vi "MapSim.vi"() -> ()   [LabVIEW 2018]
uses:
  <vilib>/imath/engines/lvmath/Plug In/_Char/NIMS_CH_character datatype.ctl
  <vilib>/Analysis/coordinate.llb/2D Cartesian Coordinate Rotation (Scalar).vi
  <vilib>/robotics/Navigation/shared/WorldMap/OccupancyGridWorldMap/NI_Robotics_OccupancyGridWorldMap.lvclass
  C:/Program Files (x86)/National Instruments/LabVIEW 2018/vi.lib/robotics/Navigation/shared/WorldMap/AbstractWorldMap/NI_Robotics_AbstractWorldMap.lvclass
  <vilib>/robotics/Navigation/shared/MapNode/OccupancyGridNode/NI_Robotics_OccupancyGridMapNode.lvclass
  C:/Program Files (x86)/National Instruments/LabVIEW 2018/vi.lib/robotics/Navigation/shared/MapNode/AbstractAstarNode/NI_Robotics_AbstractAstarNode.lvclass
  <vilib>/imath/engines/lvmath2/RunTimeEngine/Managers/WorkSpace/UID Generator.vi
  <vilib>/imath/engines/lvmath/Plug In/_Char/NIMS_CH_String to Character Array.vi
  <vilib>/imath/engines/lvmath2/RunTimeEngine/IndexRead/NIMS V(S).vi
  <instcachedir>/0/NIMS V(S)_0488751826AF41519A22953C041130DC.lvgen/NIMS V(S)_0488751826AF41519A22953C041130DC_003.vi
  <vilib>/imath/engines/lvmath2/RunTimeEngine/RunTimeType/NIMS_RunTimeType_From StrictType (excl LVString).vi
  <instcachedir>/0/NIMS_RunTimeType_From StrictType (excl LVString)_E7E34A65C99947108168652BAD14964D.lvgen/NIMS_RunTimeType_From StrictType (excl LVString)_E7E34A65C99947108168652BAD14964D_000.vi
  <vilib>/imathl/engines/lvmath/Functions/Error Handling/Create Error.vi
  <vilib>/imath/engines/lvmath2/RunTimeEngine/LocalVariableDefStatement/MC_LocalVariableDefStatement_Display.vi
  <vilib>/imath/engines/lvmath2/RunTimeEngine/BuiltInFunctions/acos/NIMS_acos(C).vi
  <instcachedir>/0/NIMS_acos(C)_EB9F8BBCD4F84158BAE4AC9B979C42E8.lvgen/NIMS_acos(C)_EB9F8BBCD4F84158BAE4AC9B979C42E8_001.vi
  <vilib>/imath/engines/lvmath2/RunTimeEngine/Managers/SymbolTable/Clear UID.vi
  <vilib>/imath/engines/lvmath2/RunTimeEngine/NodeEndStatement/NIMS_NodeEndStatement_Output.vi
  <instcachedir>/0/NIMS_NodeEndStatement_Output_53EC0D466D134D7ABD903AC30B43404B.lvgen/NIMS_NodeEndStatement_Output_53EC0D466D134D7ABD903AC30B43404B_001.vi
  <instcachedir>/0/NIMS_NodeEndStatement_Output_53EC0D466D134D7ABD903AC30B43404B.lvgen/NIMS_NodeEndStatement_Output_53EC0D466D134D7ABD903AC30B43404B_011.vi
  <instcachedir>/0/NIMS_NodeEndStatement_Output_53EC0D466D134D7ABD903AC30B43404B.lvgen/NIMS_NodeEndStatement_Output_53EC0D466D134D7ABD903AC30B43404B_009.vi
  <vilib>/imath/engines/lvmath2/RunTimeEngine/ErrorHandling/NIMS_Finalize Error.vi
  <vilib>/imath/engines/lvmath2/RunTimeEngine/BuiltInFunctions/round/NIMS_round(DBL-S).vi
  <vilib>/imath/engines/lvmath2/RunTimeEngine/BuiltInFunctions/char/NIMS_char.vi
  <vilib>/imath/engines/lvmath/Plug In/_Char/NIMS_CH_String CV to Character 2D.vi
  <instcachedir>/0/NIMS_CH_String CV to Character 2D_831D8380D97041D793313BBAC4831DC8.lvgen/NIMS_CH_String CV to Character 2D_831D8380D97041D793313BBAC4831DC8_000.vi
  <instcachedir>/0/NIMS_RunTimeType_From StrictType (excl LVString)_E7E34A65C99947108168652BAD14964D.lvgen/NIMS_RunTimeType_From StrictType (excl LVString)_E7E34A65C99947108168652BAD14964D_001.vi
  <vilib>/imath/engines/lvmath/Plug In/_Char/NIMS_CH_Character 2D to String 1D.vi
  <vilib>/imath/engines/lvmath2/RunTimeSupport/NIMS_Error if Not Equal.vi
  <instcachedir>/0/NIMS_Error if Not Equal_C77461FADD9B4AE6B0EA3ED6E3A6D94D.lvgen/NIMS_Error if Not Equal_C77461FADD9B4AE6B0EA3ED6E3A6D94D_000.vi
  <vilib>/imath/engines/lvmath2/RunTimeEngine/IndexReplace/NIMS M(S,S)=S.vi
  <instcachedir>/0/NIMS M(S,S)=S_5DAF17B45D8A4C8588C7CF468644990A.lvgen/NIMS M(S,S)=S_5DAF17B45D8A4C8588C7CF468644990A_002.vi
  <vilib>/imath/engines/lvmath2/RunTimeEngine/ErrorHandling/NIMS_Create Error From Enums.vi
  <vilib>/imath/engines/lvmath2/RunTimeEngine/RangeToken/NIMS_Range_R2 - Integer.vi
  <instcachedir>/0/NIMS_Range_R2 - Integer_E35B921DECF84AADB7325A02D418BFCC.lvgen/NIMS_Range_R2 - Integer_E35B921DECF84AADB7325A02D418BFCC_000.vi
  <vilib>/imath/engines/lvmath2/RunTimeEngine/CommandStatement/MC_CommandStatement_break.vi
  <vilib>/imath/engines/lvmath2/RunTimeEngine/BuiltInFunctions/min/2 inputs/NIMS_min(RG,RG)-no size check.vi
  <instcachedir>/0/NIMS_min(RG,RG)-no size check_7F67BAB91AFC452D9517D2EA1C8F5F88.lvgen/NIMS_min(RG,RG)-no size check_7F67BAB91AFC452D9517D2EA1C8F5F88_001.vi
  <vilib>/imath/engines/lvmath2/RunTimeEngine/BuiltInFunctions/max/2 inputs/NIMS_max(RG,RG)-no size check.vi
  <instcachedir>/0/NIMS_max(RG,RG)-no size check_F871939977644B7683C1350DCCAD7557.lvgen/NIMS_max(RG,RG)-no size check_F871939977644B7683C1350DCCAD7557_001.vi
  <vilib>/imath/engines/lvmath2/RunTimeEngine/IndexRead/NIMS M(S,S).vi
  <instcachedir>/0/NIMS M(S,S)_AC51E74150A542F7991B9634C66F3096.lvgen/NIMS M(S,S)_AC51E74150A542F7991B9634C66F3096_002.vi
  <instcachedir>/0/NIMS_min(RG,RG)-no size check_7F67BAB91AFC452D9517D2EA1C8F5F88.lvgen/NIMS_min(RG,RG)-no size check_7F67BAB91AFC452D9517D2EA1C8F5F88_002.vi
  <instcachedir>/0/NIMS_min(RG,RG)-no size check_7F67BAB91AFC452D9517D2EA1C8F5F88.lvgen/NIMS_min(RG,RG)-no size check_7F67BAB91AFC452D9517D2EA1C8F5F88_003.vi
  <vilib>/imath/engines/lvmath2/RunTimeEngine/VariableToken/NIMS_VariableToken_CondDefined.vi
  <instcachedir>/0/NIMS_VariableToken_CondDefined_BADDB804EBCA4B86883699DABD34B224.lvgen/NIMS_VariableToken_CondDefined_BADDB804EBCA4B86883699DABD34B224_004.vi
  <vilib>/imath/engines/lvmath/Functions/Error Handling/MergeErrorsWrapper.vi
  <instcachedir>/0/NIMS_NodeEndStatement_Output_53EC0D466D134D7ABD903AC30B43404B.lvgen/NIMS_NodeEndStatement_Output_53EC0D466D134D7ABD903AC30B43404B_012.vi
  <instcachedir>/0/NIMS_NodeEndStatement_Output_53EC0D466D134D7ABD903AC30B43404B.lvgen/NIMS_NodeEndStatement_Output_53EC0D466D134D7ABD903AC30B43404B_013.vi
  <instcachedir>/0/NIMS_NodeEndStatement_Output_53EC0D466D134D7ABD903AC30B43404B.lvgen/NIMS_NodeEndStatement_Output_53EC0D466D134D7ABD903AC30B43404B_016.vi
  <vilib>/imath/engines/lvmath2/RunTimeEngine/Managers/SymbolTable/NIMS_WorkSpace.lvlib
  <vilib>/Analysis/NI_AALPro.lvlib
  <vilib>/robotics/Navigation/NI_Robotics_Navigation .lvlib
panel:
  out "y coordinates":i32[](array[numeric])
  out "x coordinates":i32[](array[numeric])
  out "dy":dbl
  out "dx":dbl
  out "G":i32[][](array[numeric])
  out "dx_char":string[](array[string])
  out "dy_char":string[](array[string])
  in  "QR Data":string
  out "Field":u8[][](array[numeric])
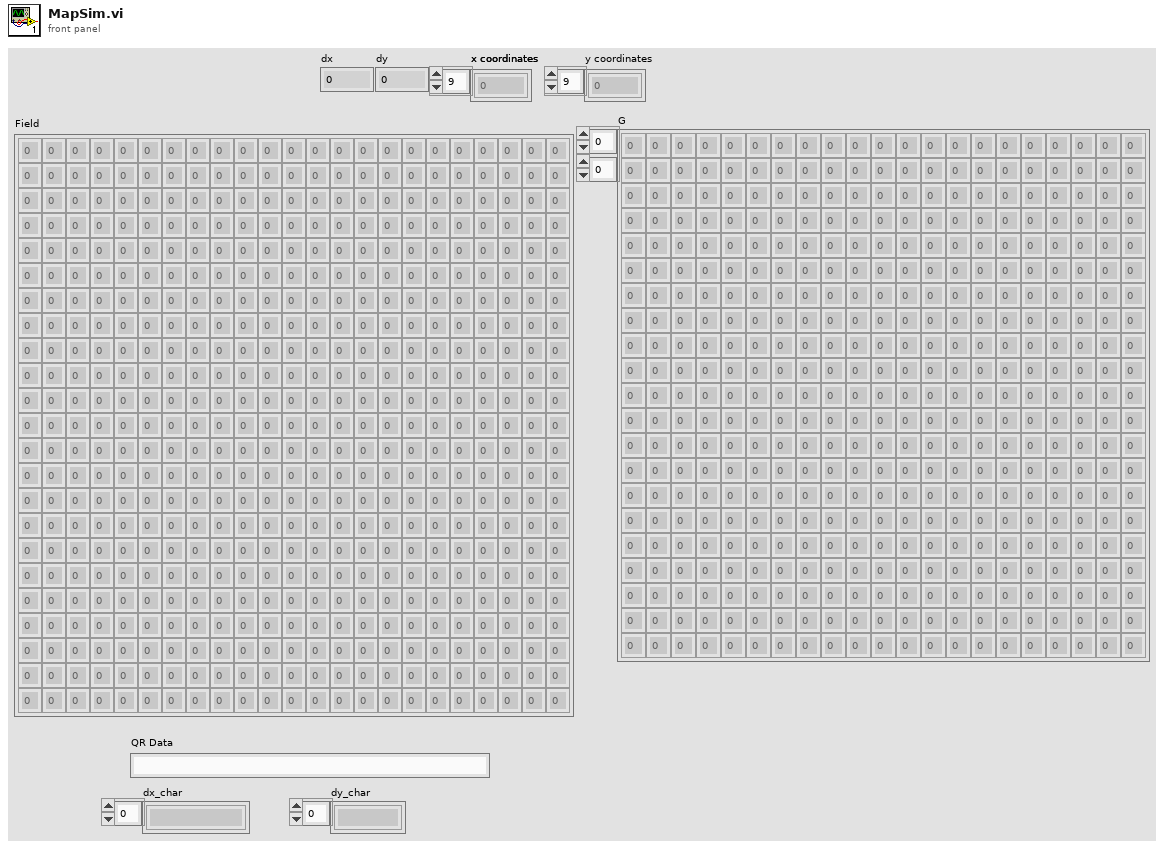
[diagram p1: front panel]
types:
  T1 = typedef "NIMS_CH_character datatype.ctl" = cluster{"Numeric":u8}
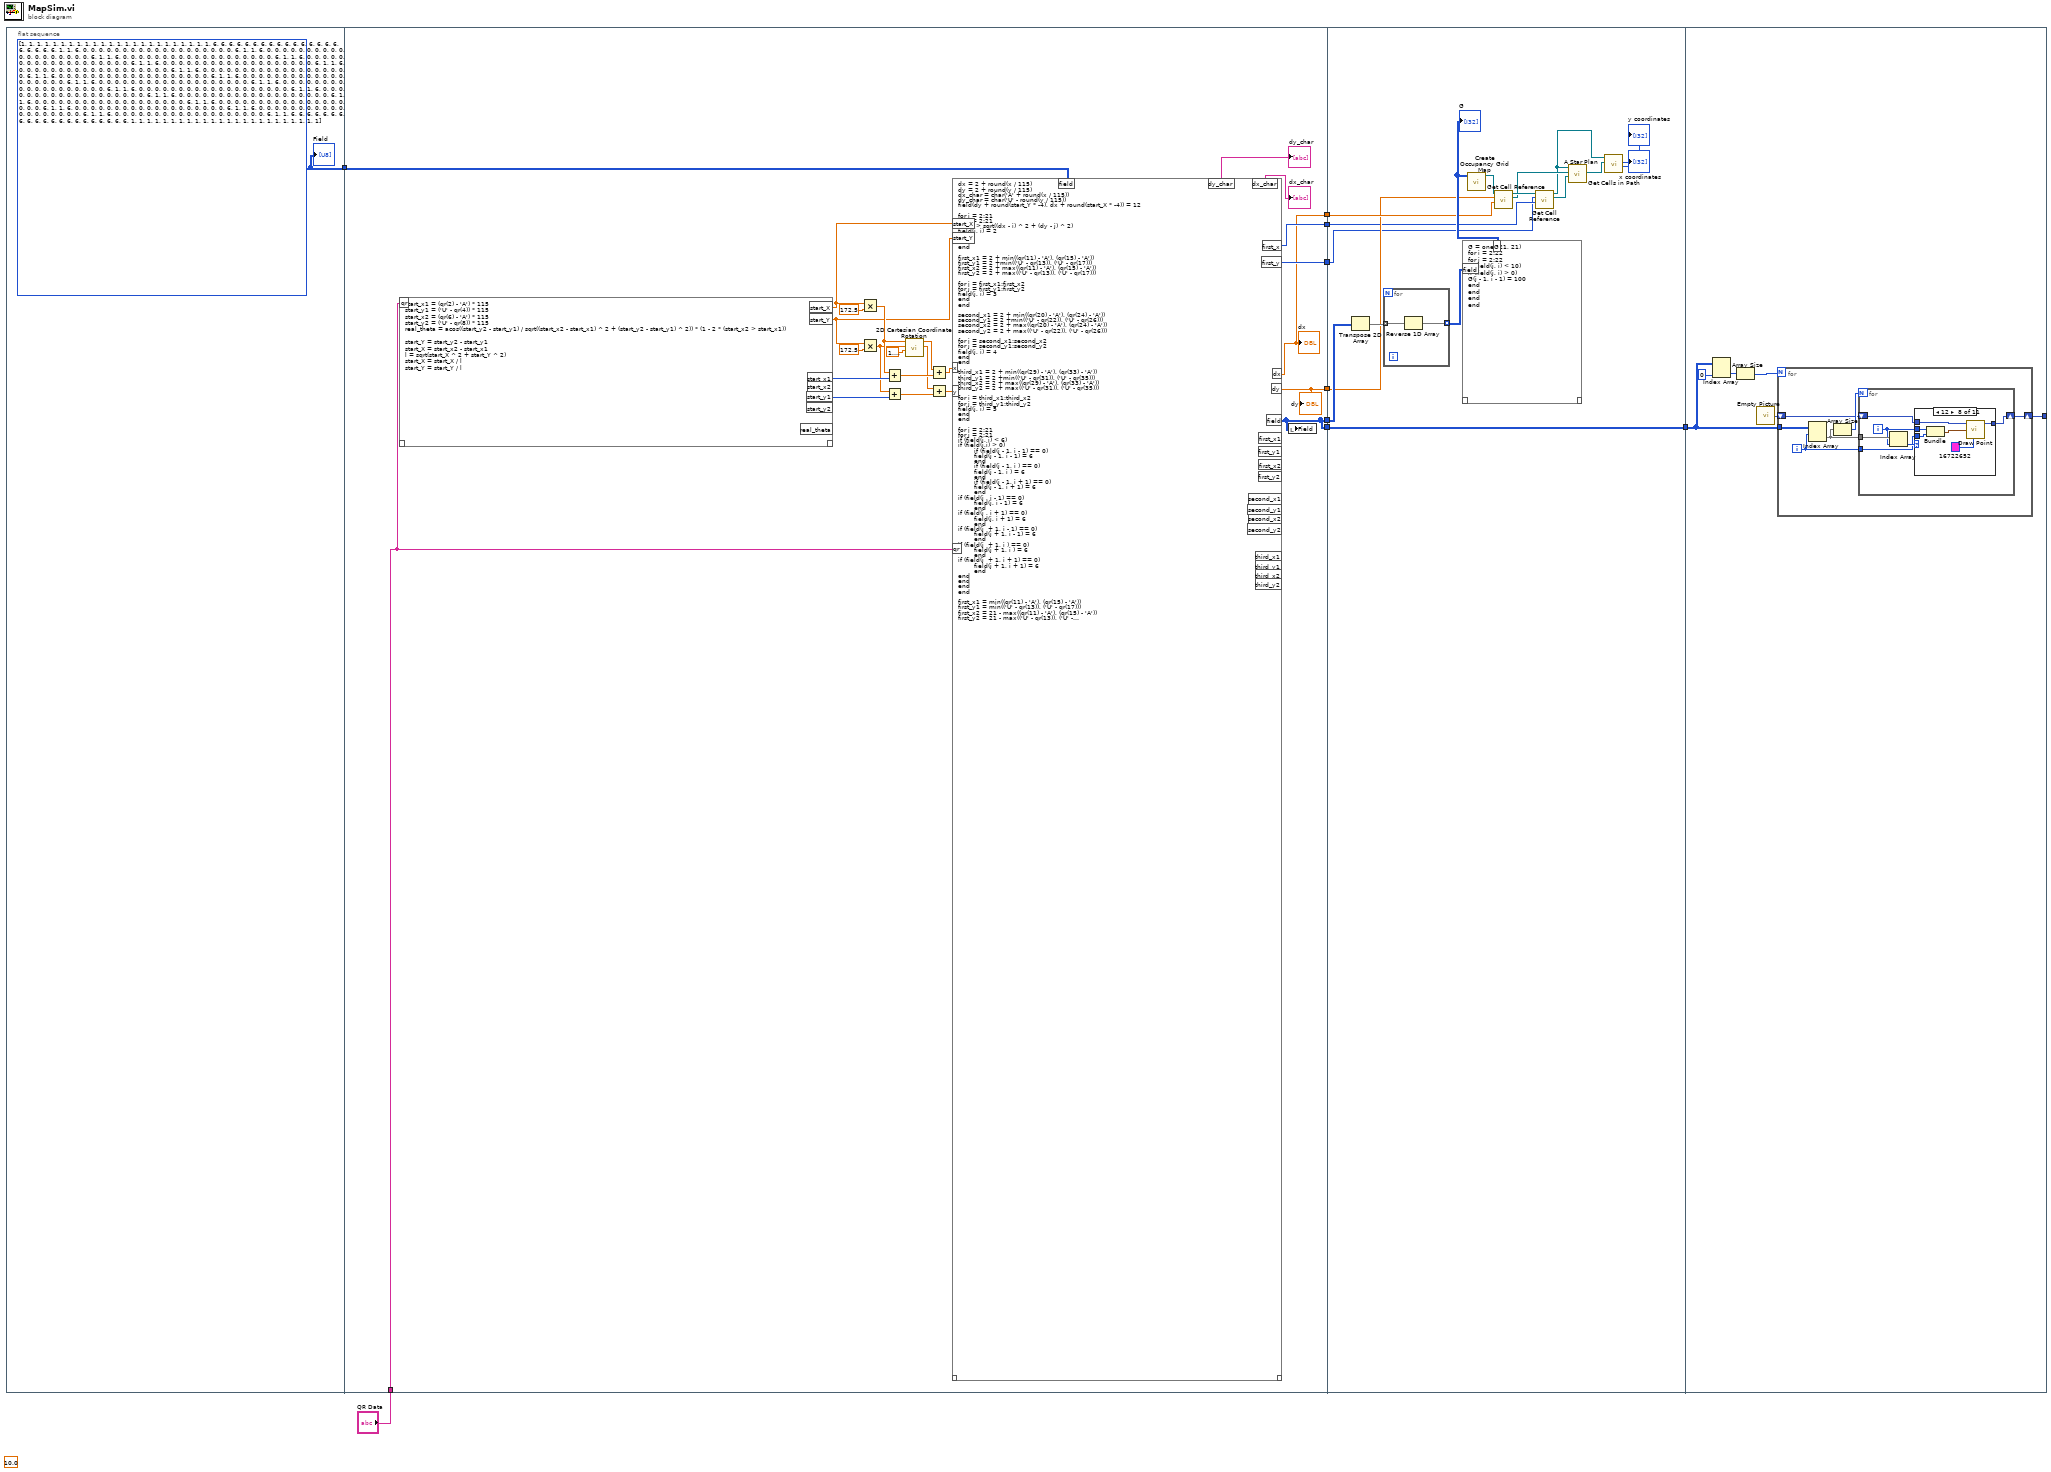
[diagram p0: block diagram]
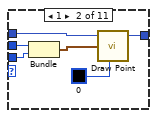
[diagram p3: hidden frame]
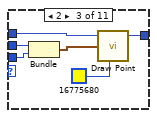
[diagram p4: hidden frame]
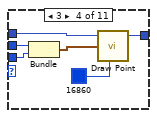
[diagram p5: hidden frame]
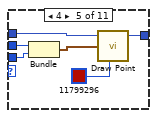
[diagram p6: hidden frame]
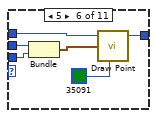
[diagram p7: hidden frame]
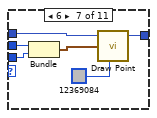
[diagram p8: hidden frame]
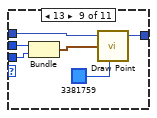
[diagram p9: hidden frame]
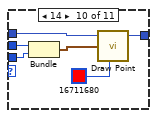
[diagram p10: hidden frame]
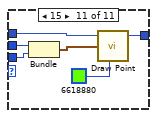
[diagram p11: hidden frame]
diagram:
  (unwired) sgl 10.0 ("Zoom Factor")
  n1 = flat-sequence {
    tunnel: [w10] -> w8
    tunnel: "QR Data" -> [w21]
    tunnel: w8 -> [w20]
    tunnel: [w15] -> w7
    tunnel: [w15] -> w5
    tunnel: [w14] -> w4
    tunnel: [w13] -> w3
    tunnel: [w12] -> w2
    tunnel: [w11] -> w1
    tunnel: w7 -> [w3612]
    tunnel: [w3612] -> w6
    tunnel: w5 -> [w3616]
    tunnel: w4 -> [w3601]
    tunnel: w3 -> [w3600]
    tunnel: w2 -> [w3603]
    tunnel: w1 -> [w3602]
    tunnel: w6 -> [w3830]
    tunnel: [w3826] -> _
    frame #0 {
      w10 = u8[][] [[1, 1, 1, 1, 1, 1, 1, 1, 1, 1, 1, 1, 1, 1, 1, 1, 1, 1, 1, 1, 1, 1, 1], [1, 6, 6, 6, 6, 6, 6, 6, 6, 6, 6, 6, 6, 6, 6, 6, 6, 6, 6, 6, 6, 6, 1], [1, 6, 0, 0, 0, 0, 0, 0, 0, 0, 0, 0, 0, 0, 0, 0, 0, 0, 0, 0, 0, 6, 1], [1, 6, 0, 0, 0, 0, 0, 0, 0, 0, 0, 0, 0, 0, 0, 0, 0, 0, 0, 0, 0, 6, 1], [1, 6, 0, 0, 0, 0, 0, 0, 0, 0, 0, 0, 0, 0, 0, 0, 0, 0, 0, 0, 0, 6, 1], [1, 6, 0, 0, 0, 0, 0, 0, 0, 0, 0, 0, 0, 0, 0, 0, 0, 0, 0, 0, 0, 6, 1], [1, 6, 0, 0, 0, 0, 0, 0, 0, 0, 0, 0, 0, 0, 0, 0, 0, 0, 0, 0, 0, 6, 1], [1, 6, 0, 0, 0, 0, 0, 0, 0, 0, 0, 0, 0, 0, 0, 0, 0, 0, 0, 0, 0, 6, 1], [1, 6, 0, 0, 0, 0, 0, 0, 0, 0, 0, 0, 0, 0, 0, 0, 0, 0, 0, 0, 0, 6, 1], [1, 6, 0, 0, 0, 0, 0, 0, 0, 0, 0, 0, 0, 0, 0, 0, 0, 0, 0, 0, 0, 6, 1], [1, 6, 0, 0, 0, 0, 0, 0, 0, 0, 0, 0, 0, 0, 0, 0, 0, 0, 0, 0, 0, 6, 1], [1, 6, 0, 0, 0, 0, 0, 0, 0, 0, 0, 0, 0, 0, 0, 0, 0, 0, 0, 0, 0, 6, 1], [1, 6, 0, 0, 0, 0, 0, 0, 0, 0, 0, 0, 0, 0, 0, 0, 0, 0, 0, 0, 0, 6, 1], [1, 6, 0, 0, 0, 0, 0, 0, 0, 0, 0, 0, 0, 0, 0, 0, 0, 0, 0, 0, 0, 6, 1], [1, 6, 0, 0, 0, 0, 0, 0, 0, 0, 0, 0, 0, 0, 0, 0, 0, 0, 0, 0, 0, 6, 1], [1, 6, 0, 0, 0, 0, 0, 0, 0, 0, 0, 0, 0, 0, 0, 0, 0, 0, 0, 0, 0, 6, 1], [1, 6, 0, 0, 0, 0, 0, 0, 0, 0, 0, 0, 0, 0, 0, 0, 0, 0, 0, 0, 0, 6, 1], [1, 6, 0, 0, 0, 0, 0, 0, 0, 0, 0, 0, 0, 0, 0, 0, 0, 0, 0, 0, 0, 6, 1], [1, 6, 0, 0, 0, 0, 0, 0, 0, 0, 0, 0, 0, 0, 0, 0, 0, 0, 0, 0, 0, 6, 1], [1, 6, 0, 0, 0, 0, 0, 0, 0, 0, 0, 0, 0, 0, 0, 0, 0, 0, 0, 0, 0, 6, 1], [1, 6, 0, 0, 0, 0, 0, 0, 0, 0, 0, 0, 0, 0, 0, 0, 0, 0, 0, 0, 0, 6, 1], [1, 6, 6, 6, 6, 6, 6, 6, 6, 6, 6, 6, 6, 6, 6, 6, 6, 6, 6, 6, 6, 6, 1], [1, 1, 1, 1, 1, 1, 1, 1, 1, 1, 1, 1, 1, 1, 1, 1, 1, 1, 1, 1, 1, 1, 1]] ("Field")
      "Field" <- w10
    }
    frame #1 {
      n2 = mathscript code="start_x1 = (qr(2) - 'A') * 115\nstart_y1 = ('U' - qr(4)) * 115\nstart_x2 = (qr(6) - 'A') * 115\nstart_y2 = ('U' - qr(8)) * 115\nreal_theta = acos((start_y2 - start_y1) / sqrt((start_x2 - start_x1) ^ 2 + (start_y2 - start_y1) ^ 2)) * (1 - 2 * (start_x2 > start_x1))\n\nstart_Y = start_y2 - start_y1\nstart_X = start_x2 - start_x1\nl = sqrt(start_X ^ 2 + start_Y ^ 2)\nstart_X = start_X / l\nstart_Y = start_Y / l"("qr"=w21) -> ("start_x1"=w34:i32, "start_y1"=w33:i32, "start_X"=w17:dbl, "start_Y"=w16:dbl)  [unwired: 1 in, 4 out]
      n3 = Multiply(x=w17, y=172.5) -> (x*y=w30:dbl)
      n4 = Multiply(x=w16, y=172.5) -> (x*y=w29:dbl)
      n5 = Add(x=w30, y=w34) -> (x+y=w28:dbl)
      n6 = Add(x=w29, y=w33) -> (x+y=w25:dbl)
      n7 = call-poly <vilib>:"2D Cartesian Coordinate Rotation.vi"("theta"=1.5707963267948966, "y"=w29, "x"=w30) -> ("y out"=w24:dbl, "x out"=w27:dbl)  [unwired: 6 in, 1 out]
      n8 = Add(x=w27, y=w28) -> (x+y=w26:dbl)
      n9 = Add(x=w24, y=w25) -> (x+y=w23:dbl)
      n10 = mathscript code="dx = 2 + round(x / 115)\ndy = 2 + round(y / 115)\ndx_char = char('A' + round(x / 115))\ndy_char = char('U' - round(y / 115))\nfield(dy + round(start_Y * -4), dx + round(start_X * -4)) = 12\n\nfor i = 2:21\nfor j = 2:21\nif 2.3 > sqrt((dx - i) ^ 2 + (dy - j) ^ 2)\nfield(j, i) = 2\nend\nend\nend\n\nfirst_x1 = 2 + min((qr(11) - 'A'), (qr(15) - 'A'))\nfirst_y1 = 2 +min(('U' - qr(13)), ('U' - qr(17)))\nfirst_x2 = 2 + max((qr(11) - 'A'), (qr(15) - 'A'))\nfirst_y2 = 2 + max(('U' - qr(13)), ('U' - qr(17)))\n\nfor i = first_x1:first_x2\nfor j = first_y1:first_y2\nfield(j, i) = 3\nend\nend\n\nsecond_x1 = 2 + min((qr(20) - 'A'), (qr(24) - 'A'))\nsecond_y1 = 2 +min(('U' - qr(22)), ('U' - qr(26)))\nsecond_x2 = 2 + max((qr(20) - 'A'), (qr(24) - 'A'))\nsecond_y2 = 2 + max(('U' - qr(22)), ('U' - qr(26)))\n\nfor i = second_x1:second_x2\nfor j = second_y1:second_y2\nfield(j, i) = 4\nend\nend\n\nthird_x1 = 2 + min((qr(29) - 'A'), (qr(33) - 'A'))\nthird_y1 = 2 +min(('U' - qr(31)), ('U' - qr(35)))\nthird_x2 = 2 + max((qr(29) - 'A'), (qr(33) - 'A'))\nthird_y2 = 2 + max(('U' - qr(31)), ('U' - qr(35)))\n\nfor i = third_x1:third_x2\nfor j = third_y1:third_y2\nfield(j, i) = 5\nend\nend\n\nfor i = 2:21\nfor j = 2:21\nif (field(j, i) < 6)\nif (field(j,i) > 0)\n        if (field(j - 1, i - 1) == 0)\n        field(j - 1, i - 1) = 6\n        end\n        if (field(j - 1, i ) == 0)\n        field(j - 1, i ) = 6\n        end\n        if (field(j - 1, i + 1) == 0)\n        field(j - 1, i + 1) = 6\n        end\nif (field(j , i - 1) == 0)\n        field(j, i - 1) = 6\n        end\nif (field(j , i + 1) == 0)\n        field(j, i + 1) = 6\n        end\nif (field(j  + 1, i - 1) == 0)\n        field(j + 1, i - 1) = 6\n        end\nif (field(j  + 1, i ) == 0)\n        field(j + 1, i ) = 6\n        end\nif (field(j  + 1, i + 1) == 0)\n        field(j + 1, i + 1) = 6\n        end\nend\nend\nend\nend\n\nfirst_x1 = min((qr(11) - 'A'), (qr(15) - 'A'))\nfirst_y1 = min(('U' - qr(13)), ('U' - qr(17)))\nfirst_x2 = 21 - max((qr(11) - 'A'), (qr(15) - 'A'))\nfirst_y2 = 21 - max(('U' - qr(13)), ('U' - qr(17)))\n\nmin_dist = min(first_x1, min(first_x2, min(first_y1, first_y2)))\nif min_dist == first_x1\n    field(2 + first_y1 + 1, 2 + 21 -first_x2 + 2) = 13\nfirst_x = 21 -first_x2 + 2\nfirst_y = first_y1 + 1\nend\nif min_dist == first_x2\n    field(2 + first_y1 + 1, 2 + first_x1 - 2) = 13\nfirst_x = first_x1 - 2\nfirst_y = first_y1 + 1\nend\nif min_dist == first_y1\n    field(2 + 21 - first_y2 + 2, 2 + first_x1 + 1) = 13\nfirst_x = first_x1 + 1\nfirst_y = 21 - first_y2 + 2\nend\nif min_dist == first_y2\n    field(2 + first_y1 - 2, 2 + first_x1 + 1) = 13\nfirst_x =  first_x1 + 1\nfirst_y = first_y1 - 2\nend\n\n\n\nfirst_x1 = min((qr(20) - 'A'), (qr(24) - 'A'))\nfirst_y1 = min(('U' - qr(22)), ('U' - qr(26)))\nfirst_x2 = 21 - max((qr(20) - 'A'), (qr(24) - 'A'))\nfirst_y2 = 21 - max(('U' - qr(22)), ('U' - qr(26)))\n\nmin_dist = min(first_x1, min(first_x2, min(first_y1, first_y2)))\nif min_dist == first_x1\n    field(2 + first_y1 + 1, 2 + 21 -first_x2 + 2) = 14\nend\nif min_dist == first_x2\n    field(2 + first_y1 + 1, 2 + first_x1 - 2) = 14\nend\nif min_dist == first_y1\n    field(2 + 21 - first_y2 + 2, 2 + first_x1 + 1) = 14\nend\nif min_dist == first_y2\n    field(2 + first_y1 - 2, 2 + first_x1 + 1) = 14\nend\n\nfirst_x1 = min((qr(29) - 'A'), (qr(33) - 'A'))\nfirst_y1 = min(('U' - qr(31)), ('U' - qr(35)))\nfirst_x2 = 21 - max((qr(29) - 'A'), (qr(33) - 'A'))\nfirst_y2 = 21 - max(('U' - qr(31)), ('U' - qr(35)))\n\nmin_dist = min(first_x1, min(first_x2, min(first_y1, first_y2)))\nif min_dist == first_x1\n    field(2 + first_y1 + 1, 2 + 21 -first_x2 + 2) = 15\nend\nif min_dist == first_x2\n    field(2 + first_y1 + 1, 2 + first_x1 - 2) = 15\nend\nif min_dist == first_y1\n    field(2 + 21 - first_y2 + 2, 2 + first_x1 + 1) = 15\nend\nif min_dist == first_y2\n    field(2 + first_y1 - 2, 2 + first_x1 + 1) = 15\nend\n\ndx  = dx + round(start_X * -4) - 2\ndy = dy + round(start_Y * -4) - 2"("x"=w26, "y"=w23, "field"=w20, "qr"=w21, "start_X"=w17, "start_Y"=w16) -> ("dx"=w12:dbl, "dy"=w11:dbl, "field"=w15:i32[][], "dx_char"=→"dx_char":string[], "dy_char"=→"dy_char":string[], "first_x"=w14:i32, "first_y"=w13:i32)  [unwired: 1 in, 13 out]
      "dx" <- w12
      "dy" <- w11
      n11 = local write "Field"(w15) -> ()
    }
    frame #2 {
      n12 = Transpose 2D Array(2D array=w3616) -> (transposed array=w3615:i32[][])
      n13 = for {
        tunnel: w3615 -> [w3825] mode=indexing
        tunnel: [w3824] -> w3614 mode=indexing
        n14 = Reverse 1D Array(array=w3825) -> (reversed array=w3824:i32[])
      }
      n15 = mathscript code="G = ones(21, 21)\nfor i = 2:22\nfor j = 2:22\nif (field(j, i) < 10)\nif (field(j, i) > 0)\nG(j - 1, i - 1) = 100\nend\nend\nend\nend"("field"=w3614) -> ("G"=w3613:i32[][])  [unwired: 1 in, 1 out]
      "G" <- w3613
      n16 = call <vilib>:"Create Occupancy Grid Map.vi"("occupancy grid"=w3613) -> ("map reference out"=w3611:refnum<data-value>)  [unwired: 9 in, 1 out]
      n17 = call <vilib>:"Get Cell Reference.vi"("y"=w3603, "x"=w3602, "map reference in"=w3611) -> ("cell reference"=w3609:refnum<data-value>, "map reference out"=w3610:refnum<data-value>)  [unwired: 5 in, 2 out]
      n18 = call <vilib>:"Get Cell Reference.vi"("y"=w3601, "x"=w3600, "map reference in"=w3610) -> ("cell reference"=w3608:refnum<data-value>, "map reference out"=w3607:refnum<data-value>)  [unwired: 5 in, 2 out]
      n19 = call <vilib>:"A Star Plan.vi"("goal reference"=w3608, "start reference"=w3609, "map reference in"=w3607) -> ("path references"=w3606:refnum<data-value>[])  [unwired: 5 in, 3 out]
      n20 = call <vilib>:"Get Cells in Path.vi"("path references"=w3606, "map reference in"=w3607) -> ("y coordinates"=→"y coordinates":i32[], "x coordinates"=→"x coordinates":i32[])  [unwired: 6 in, 2 out]
    }
    frame #3 {
      n21 = Index Array(array=w3830, index (col)=0 ("disabled index (col)")) -> (element=w3828:i32[])  [unwired: 1 in]
      n22 = Array Size(array=w3828) -> (size(s)=w3827:i32)
      n23 = call "Empty Picture"() -> ("empty picture"=w3831:picture)
      n24 = for {
        N: w3827 -> [_]
        tunnel: w3830 -> [w3837]
        shift-right: [w3832] -> w3826
        shift-left: w3831 -> [w3834]
        i -> [w3833]
        n25 = Index Array(array=w3837, index (row)=w3833) -> (element=w3835:i32[])  [unwired: 1 in]
        n26 = Array Size(array=w3835) -> (size(s)=w3836:i32)
        n27 = for {
          N: w3836 -> [_]
          tunnel: w3835 -> [w3843]
          tunnel: w3833 -> [w3839]
          shift-right: [w3838] -> w3832
          shift-left: w3834 -> [w3841]
          i -> [w3840]
          n28 = Index Array(array=w3843, index=w3840) -> (element=w3842:i32)
          n29 = case shown="12" w3842 {
            tunnel: w3841 -> [w3844 w3846 w3852 w3858 w3864 w3873 w3880 w3885 w3890 w3896 w3901]
            tunnel: w3840 -> [_ w3848 w3853 w3861 w3867 w3871 w3879 w3883 w3889 w3895 w3900]
            tunnel: w3839 -> [_ w3847 w3854 w3860 w3866 w3870 w3878 w3882 w3888 w3894 w3899]
            tunnel: [w3844 w3845 w3851 w3857 w3863 w3869 w3875 w3884 w3887 w3897 w3903] -> w3838
            frame 0, Default {
            }
            frame 1 {
              n30 = Bundle(w3848, w3847) -> (w3850:cluster{i32, i32})  [unwired: 1 in]
              n31 = call <vilib>:"Draw Point.vi"("picture"=w3846, "point(x,y)"=w3850, "color(black)"=u32 0) -> ("new picture"=w3845:picture)  [unwired: 6 in]
            }
            frame 2 {
              n32 = Bundle(w3853, w3854) -> (w3856:cluster{i32, i32})  [unwired: 1 in]
              n33 = call <vilib>:"Draw Point.vi"("picture"=w3852, "point(x,y)"=w3856, "color(black)"=u32 16775680) -> ("new picture"=w3851:picture)  [unwired: 6 in]
            }
            frame 3 {
              n34 = Bundle(w3861, w3860) -> (w3859:cluster{i32, i32})  [unwired: 1 in]
              n35 = call <vilib>:"Draw Point.vi"("picture"=w3858, "point(x,y)"=w3859, "color(black)"=u32 16860) -> ("new picture"=w3857:picture)  [unwired: 6 in]
            }
            frame 4 {
              n36 = Bundle(w3867, w3866) -> (w3865:cluster{i32, i32})  [unwired: 1 in]
              n37 = call <vilib>:"Draw Point.vi"("picture"=w3864, "point(x,y)"=w3865, "color(black)"=u32 11799296) -> ("new picture"=w3863:picture)  [unwired: 6 in]
            }
            frame 5 {
              n38 = Bundle(w3871, w3870) -> (w3872:cluster{i32, i32})  [unwired: 1 in]
              n39 = call <vilib>:"Draw Point.vi"("picture"=w3873, "point(x,y)"=w3872, "color(black)"=u32 35091) -> ("new picture"=w3869:picture)  [unwired: 6 in]
            }
            frame 6 {
              n40 = Bundle(w3879, w3878) -> (w3877:cluster{i32, i32})  [unwired: 1 in]
              n41 = call <vilib>:"Draw Point.vi"("picture"=w3880, "point(x,y)"=w3877, "color(black)"=u32 12369084) -> ("new picture"=w3875:picture)  [unwired: 6 in]
            }
            frame 12 {
              n42 = Bundle(w3883, w3882) -> (w3881:cluster{i32, i32})  [unwired: 1 in]
              n43 = call <vilib>:"Draw Point.vi"("picture"=w3885, "point(x,y)"=w3881, "color(black)"=u32 16722652) -> ("new picture"=w3884:picture)  [unwired: 6 in]
            }
            frame 13 {
              n44 = Bundle(w3889, w3888) -> (w3892:cluster{i32, i32})  [unwired: 1 in]
              n45 = call <vilib>:"Draw Point.vi"("picture"=w3890, "point(x,y)"=w3892, "color(black)"=u32 3381759) -> ("new picture"=w3887:picture)  [unwired: 6 in]
            }
            frame 14 {
              n46 = Bundle(w3895, w3894) -> (w3893:cluster{i32, i32})  [unwired: 1 in]
              n47 = call <vilib>:"Draw Point.vi"("picture"=w3896, "point(x,y)"=w3893, "color(black)"=u32 16711680) -> ("new picture"=w3897:picture)  [unwired: 6 in]
            }
            frame 15 {
              n48 = Bundle(w3900, w3899) -> (w3902:cluster{i32, i32})  [unwired: 1 in]
              n49 = call <vilib>:"Draw Point.vi"("picture"=w3901, "point(x,y)"=w3902, "color(black)"=u32 6618880) -> ("new picture"=w3903:picture)  [unwired: 6 in]
            }
          }
        }
      }
    }
  }
